vi "全局变量.vi"() -> ()   [LabVIEW 2023]
panel:
  out "是否踩到雷区":bool
  out "剩余方块":u16
  out "游戏状态":bool
  out "簇":T1
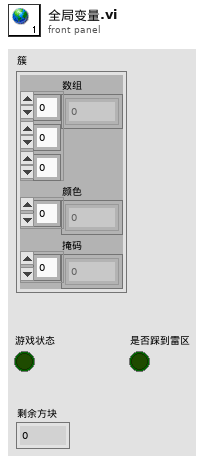
[diagram p1: front panel]
types:
  T1 = cluster{"数组":i32[][][], "colors":u32[], "mask":u8[]}
diagram:
